vi "Sort_Tracks_On_Length-2.vi"(4 "error IN":errorcluster, 5 "[IN] Min Track Length":i32, 7 "[IN] Tracks w/t Problems":T1(array[cluster])) -> (0 "error OUT":errorcluster, 1 "[OUT] Short Tracks":cluster{"Short Tracks":dbl[], "Start Pos":i32}[](array[cluster]), 3 "[OUT] Long Tracks (Filtered)":T1(array[cluster]))   [LabVIEW 2017]
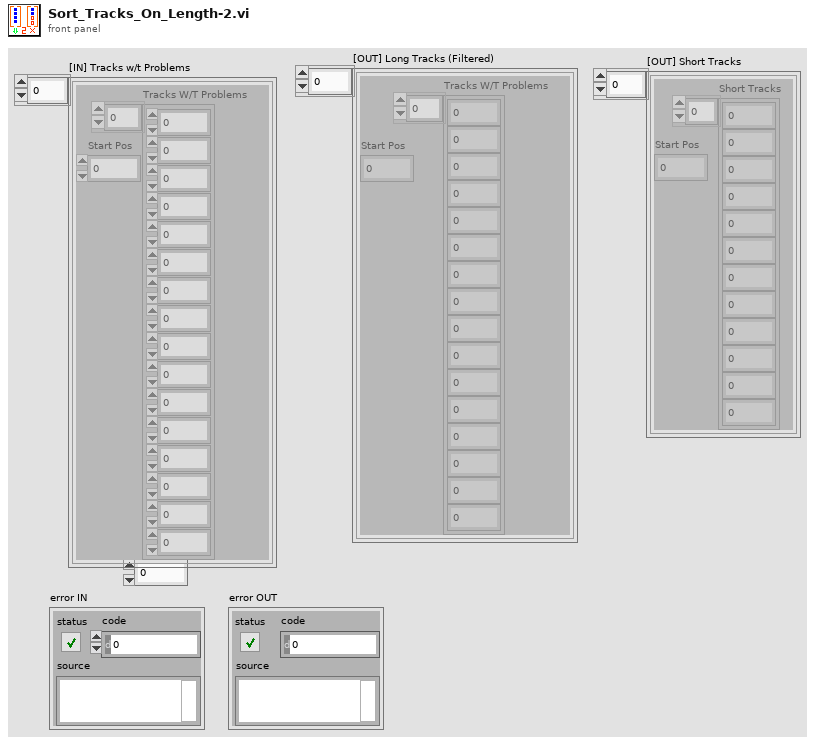
[diagram p1: front panel]
types:
  T1 = cluster{"Tracks W/T Problems":dbl[], "Start Pos":i32}[]
  T2 = cluster{"Tracks W/T Problems":dbl[], "Start Pos":i32}
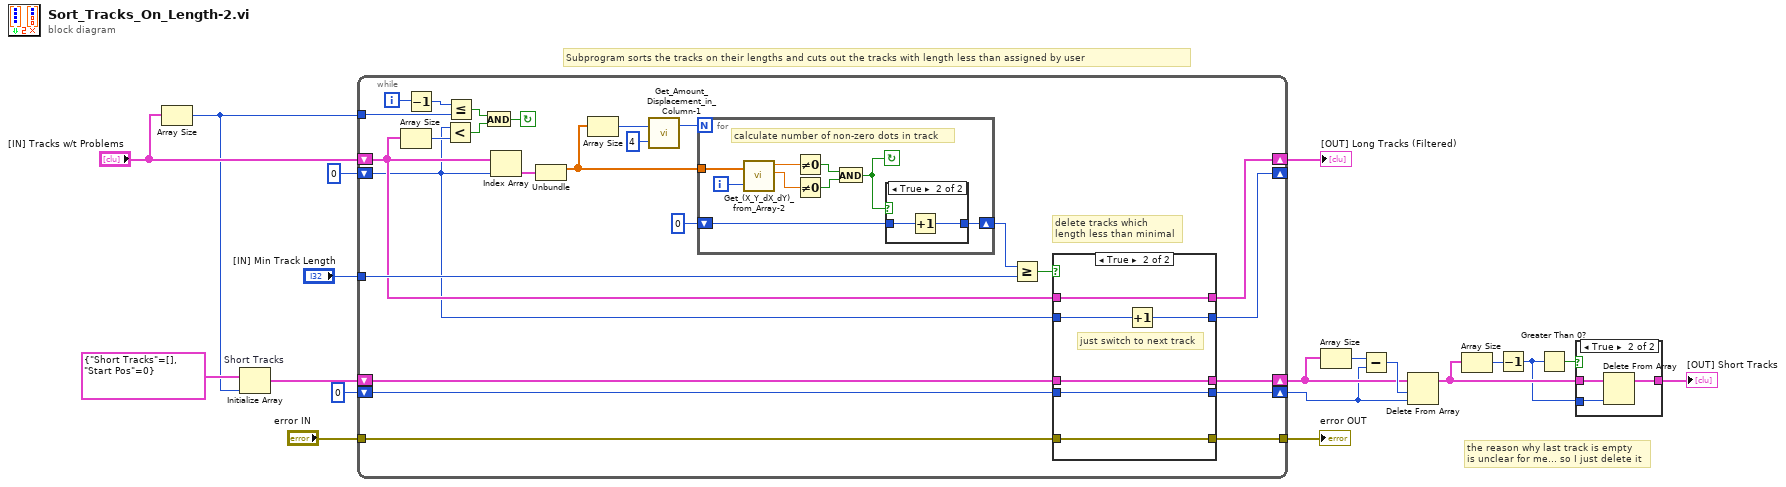
[diagram p0: block diagram]
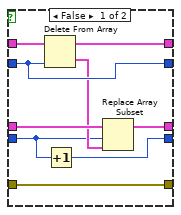
[diagram p3: hidden frame]
diagram:
  # "the reason why last track is empty \nis unclear for me... so I just delete it"
  # "Subprogram sorts the tracks on their lengths and cuts out the tracks with length less than assigned by user"
  n1 = Array Size(array="[IN] Tracks w/t Problems") -> (size(s)=w15:i32)
  n2 = Initialize Array "Short Tracks"(cluster{"Short Tracks":dbl[], "Start Pos":i32} {"Short Tracks"=[], "Start Pos"=0} ("element"), w15) -> (w14:cluster{"Short Tracks":dbl[], "Start Pos":i32}[])
  n3 = while {
    tunnel: "[IN] Min Track Length" -> [w43]
    shift-right: [w27] -> w10
    shift-left: "[IN] Tracks w/t Problems" -> [w29]
    tunnel: w15 -> [w35]
    shift-right: [w26] -> _
    shift-left: 0 -> [w28]
    shift-right: [w23] -> w7
    shift-left: w14 -> [w25]
    shift-right: [w22] -> w6
    shift-left: 0 -> [w24]
    tunnel: "error IN" -> [w21]
    tunnel: [w20] -> w11
    i -> [w36]
    stop <- w37 continue-if-true
    # "delete tracks which\nlength less than minimal"
    n4 = Array Size(array=w29) -> (size(s)=w40:i32)
    n5 = Decrement(x=w36) -> (x-1=w38:i32)
    n6 = Less?(x=w28, y=w40) -> (x < y?=w39:bool)
    n7 = Less Or Equal?(x=w38, y=w35) -> (x <= y?=w41:bool)
    n8 = And(x=w41, y=w39) -> (x .and. y?=w37:bool)
    n9 = Index Array(array=w29, index=w28) -> (element=w34:T2)
    n10 = Unbundle(w34) -> ("Tracks W/T Problems"=w30:dbl[])  [unwired: 1 out]
    n11 = Array Size(array=w30) -> (size(s)=w32:i32)
    n12 = call "Get_Amount_Displacement_in_Column-1.vi"("multiplier"=4, "# Rows"=w32) -> ("Displ amount"=w31:i32)  [unwired: 1 out]
    n13 = for {
      N: w31 -> [_]
      shift-right: [w65] -> w44
      shift-left: 0 -> [w66]
      tunnel: w30 -> [w63]
      i -> [w64]
      stop <- w67 continue-if-true
      # "calculate number of non-zero dots in track"
      n14 = call "Get_(X_Y_dX_dY)_from_Array-2.vi"("(X,Y,dX,dY)"=w63, "Index of Displacement"=w64) -> ("X"=w62:dbl, "Y"=w61:dbl)  [unwired: 2 out]
      n15 = Not Equal To 0?(x=w62) -> (x != 0?=w68:bool)
      n16 = Not Equal To 0?(x=w61) -> (x != 0?=w69:bool)
      n17 = And(x=w68, y=w69) -> (x .and. y?=w67:bool)
      n18 = case shown="True" w67 {
        tunnel: w66 -> [w70 w72]
        tunnel: [w70 w71] -> w65
        frame False {
        }
        frame True {
          n19 = Increment(x=w72) -> (x+1=w71:i32)
        }
      }
    }
    n20 = Greater Or Equal?(x=w44, y=w43) -> (x >= y?=w42:bool)
    n21 = case shown="True" w42 {
      tunnel: w29 -> [w54 w59]
      tunnel: w28 -> [w52 w60]
      tunnel: [w53 w59] -> w27
      tunnel: [w52 w58] -> w26
      tunnel: w25 -> [w51 w57]
      tunnel: w24 -> [w48 w56]
      tunnel: [w49 w57] -> w23
      tunnel: [w47 w56] -> w22
      tunnel: w21 -> [w46 w55]
      tunnel: [w46 w55] -> w20
      frame False {
        n22 = Delete From Array(array=w54, index=w52) -> (deleted portion=w50:T2, array with subset deleted=w53:T1)  [unwired: 1 in]
        n23 = Increment(x=w48) -> (x+1=w47:i32)
        n24 = Replace Array Subset(array=w51, new element=w50, index=w48) -> (w49:cluster{"Short Tracks":dbl[], "Start Pos":i32}[])
      }
      frame True {
        # "just switch to next track"
        n25 = Increment(x=w60) -> (x+1=w58:i32)
      }
    }
  }
  "error OUT" <- w11
  "[OUT] Long Tracks (Filtered)" <- w10
  n26 = Array Size(array=w7) -> (size(s)=w9:i32)
  n27 = Subtract(x=w9, y=w6) -> (x-y=w8:i32)
  n28 = Delete From Array(array=w7, length=w8, index=w6) -> (array with subset deleted=w5:cluster{"Short Tracks":dbl[], "Start Pos":i32}[])  [unwired: 1 out]
  n29 = Array Size(array=w5) -> (size(s)=w4:i32)
  n30 = Decrement(x=w4) -> (x-1=w2:i32)
  n31 = Greater Than 0?(x=w2) -> (x > 0?=w1:bool)
  n32 = case shown="True" w1 {
    tunnel: w5 -> [w73 w76]
    tunnel: [w73 w75] -> w3
    tunnel: w2 -> [_ w74]
    frame False {
    }
    frame True {
      n33 = Delete From Array(array=w76, index=w74) -> (array with subset deleted=w75:cluster{"Short Tracks":dbl[], "Start Pos":i32}[])  [unwired: 1 in, 1 out]
    }
  }
  "[OUT] Short Tracks" <- w3
